vi "getWavelength_v80_AS1_actualTime.vi"() -> ()   [LabVIEW 2016]
uses:
  <vilib>/Analysis/baseanly.llb/Mean (DBL).vi
  <vilib>/Analysis/NI_AALBase.lvlib
  x32/CLDevIFace.dll
panel:
  out "Wavelength vs. time":dbl(graph)
  out "Wavelength":dbl format="%0.5f"
  out "0.75ppm in Wave (nm)":dbl format="%#_3g"
  out "0.75ppm in Freq (MHz)":dbl
  out "Freq (Hz)":dbl
  in  "Avg":i32=1
  out "Power (mW)":dbl format="%.9f"
  in  "Delay Time (s)":dbl=0.01
  out "error out":errorcluster
  out "output param":i32
  in  "stop":bool
  in  "OK Button":bool
  in  "CommPort":dbl=5.0 caption="Comm Port #"
  # "Pr = 605.977 nm"
  # "Super cavity FSR  6 GHz\nZerodure FSR  750 MHz"
  # "1 pm = 200 MHz @1212nm\n1 pm = 800 MHz @606 nm"
  # "Bristol 621B accuracy = 0.75 ppm\nuseful conversions:"
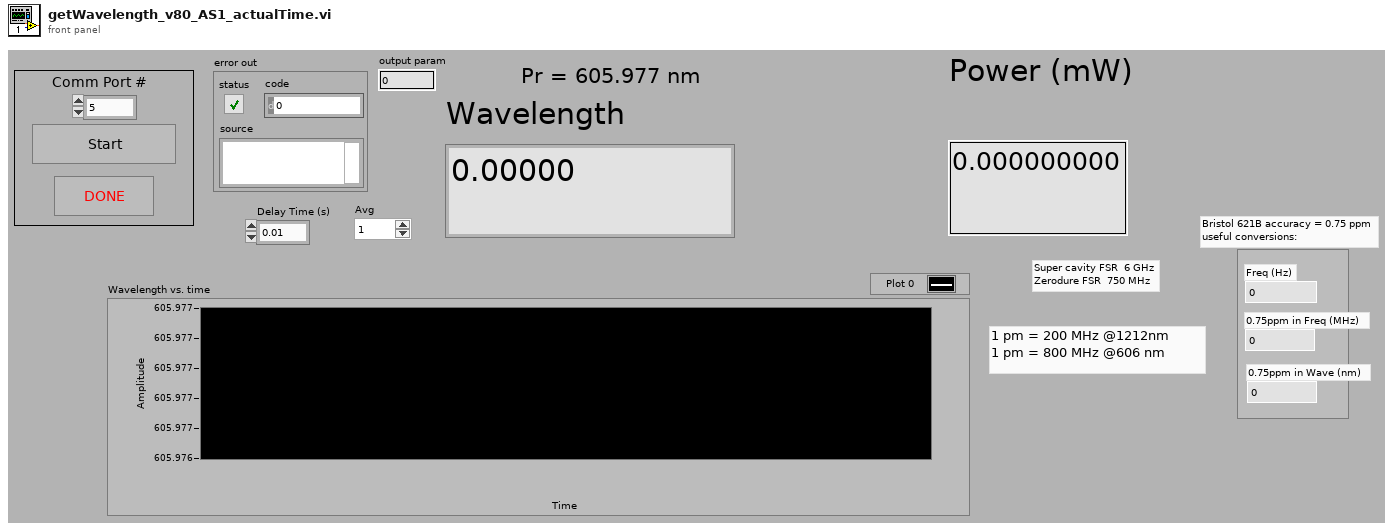
[diagram p1: front panel]
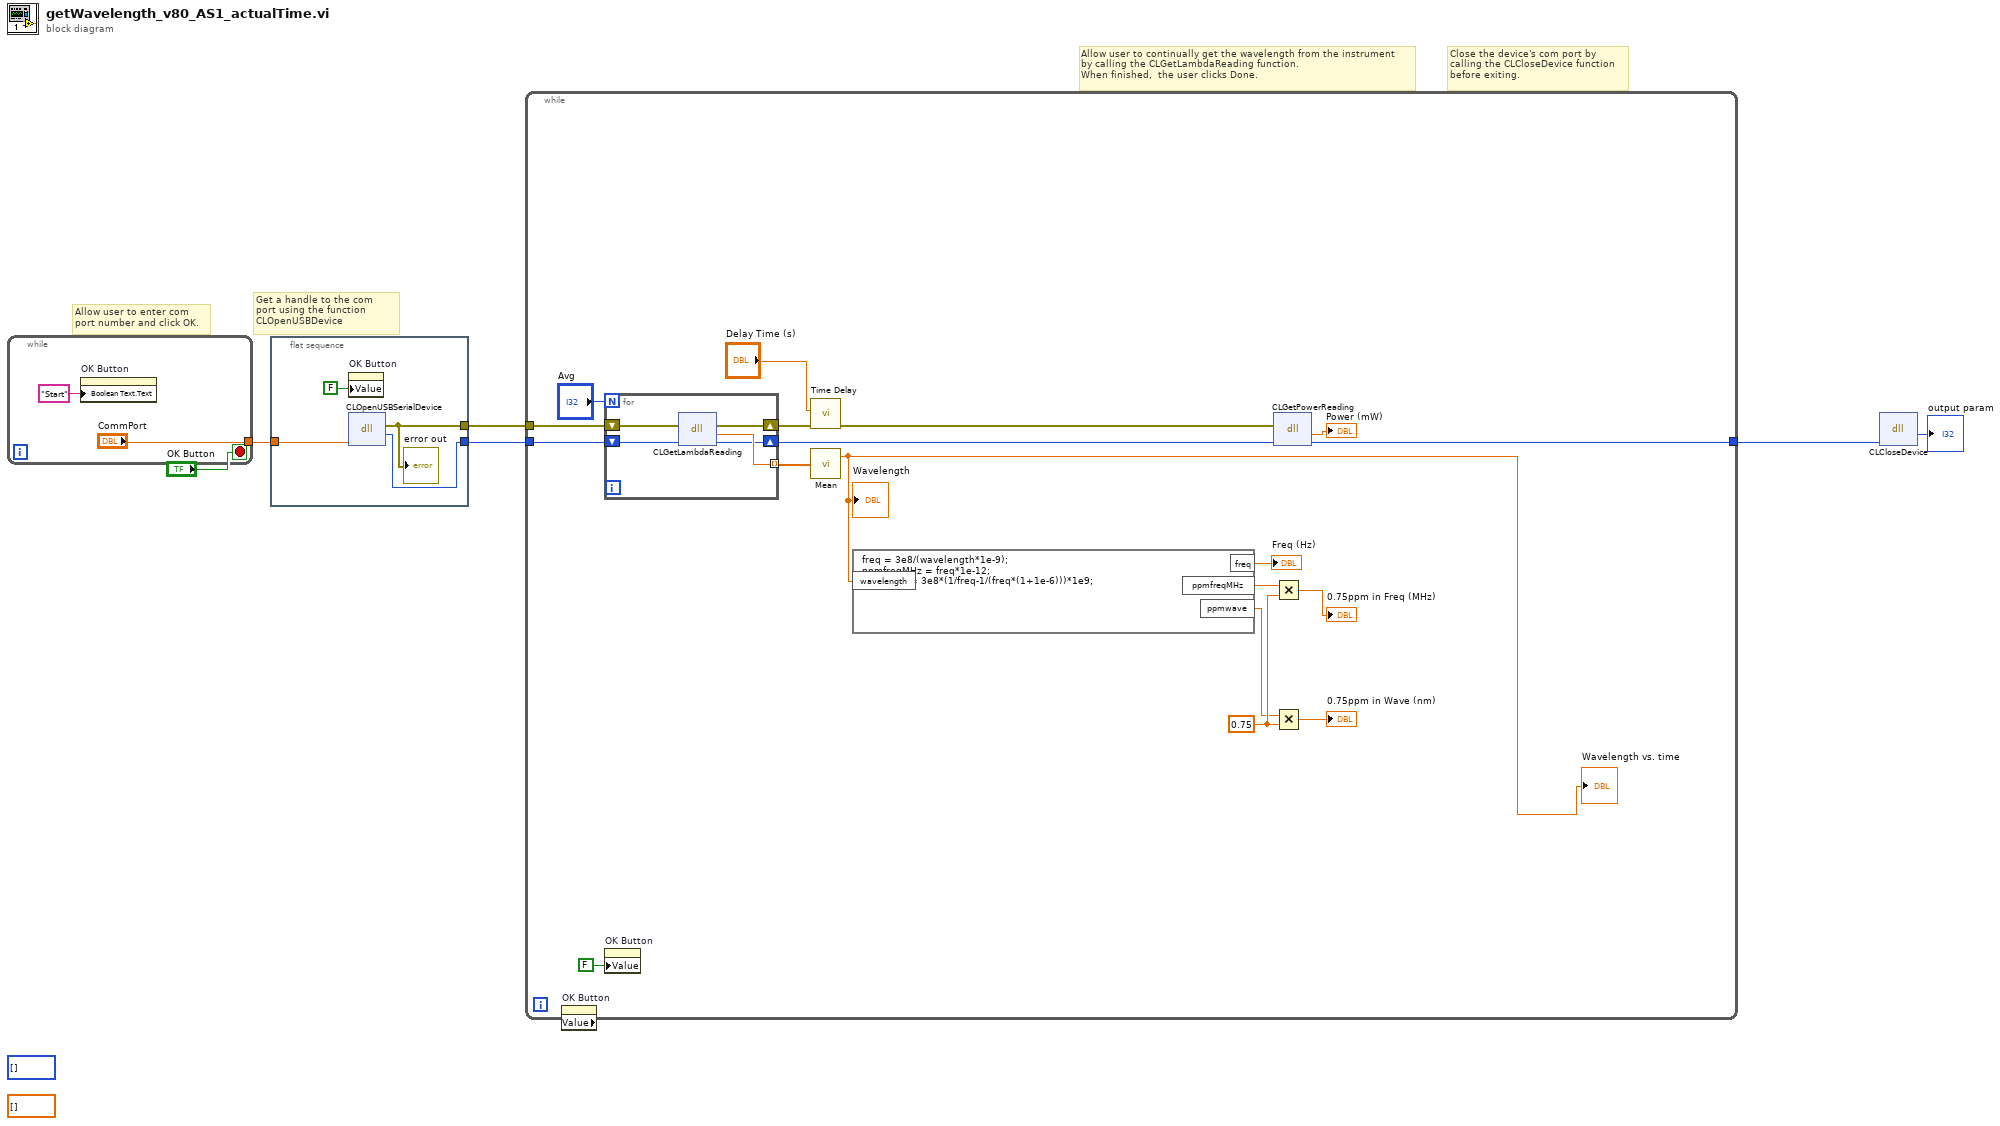
[diagram p0: block diagram]
diagram:
  (unwired) i32[] []
  (unwired) dbl[] []
  # "Close the device's com port by\ncalling the CLCloseDevice function\nbefore exiting."
  # "Allow user to continually get the wavelength from the instrument\nby calling the CLGetLambdaReading function.  \nWhen finished,  the user clicks Done."
  # "Get a handle to the com\nport using the function CLOpenUSBDevice"
  # "Allow user to enter com \nport number and click OK."
  n1 = while {
    tunnel: ["CommPort"] -> w5
    stop <- "OK Button" stop-if-true
    n2 = property on="OK Button" class="Bool (strict)"("Boolean Text.Text"="Start") -> ()  [unwired: 2 in, 2 out]
  }
  n3 = flat-sequence {
    tunnel: w5 -> [w12]
    tunnel: [w11] -> w4
    tunnel: [w9] -> w1
    frame #0 {
      n4 = property on="OK Button" class="Bool (strict)"("Value"=FALSE) -> ()  [unwired: 2 in, 2 out]
      n5 = dll-call lib="C:/Users/Lab/Desktop/Bristol wavemeter 621/00424-2-00 621 customer CD/Programming Interface/x32/CLDevIFace.dll" fn="CLOpenUSBSerialDevice"("commPort"=w12) -> (error out=w9:errorcluster, "return type"=w11:i32)  [unwired: 4 in, 1 out]
      "error out" <- w9
    }
  }
  n6 = while {
    tunnel: w4 -> [w31]
    tunnel: [w22] -> w3
    tunnel: w1 -> [w26]
    stop <- "stop" stop-if-true
    w16 = 0.75 ("y")
    n7 = property on="OK Button" class="Bool (strict)" props=["Value"]() -> ()  [unwired: 2 in, 3 out]
    n8 = for {
      N: "Avg" -> [_]
      tunnel: [w35] -> w20 mode=indexing
      shift-right: [w32] -> w23
      shift-left: w31 -> [w36]
      shift-right: [w34] -> w27
      shift-left: w26 -> [w33]
      n9 = dll-call lib="C:/Users/Lab/Desktop/Bristol wavemeter 621/00424-2-00 621 customer CD/Programming Interface/x32/CLDevIFace.dll" fn="CLGetLambdaReading"(error in=w33, "devHandle"=w36) -> (error out=w34:errorcluster, "return type"=w35:dbl, "devHandle"=w32:i32)  [unwired: 2 in, 1 out]
    }
    n10 = property on="OK Button" class="Bool (strict)"("Value"=FALSE) -> ()  [unwired: 2 in, 2 out]
    n11 = call "Time Delay"("error in (no error)"=w27, "Delay Time (s)"="Delay Time (s)") -> ("error out"=w25:errorcluster)  [unwired: 9 in]
    n12 = call-poly <vilib>:"Mean.vi"("X"=w20) -> ("mean"=w13:dbl)  [unwired: 1 out]
    "Wavelength" <- w13
    "Wavelength vs. time" <- w13
    n13 = formula code="freq = 3e8/(wavelength*1e-9);\nppmfreqMHz = freq*1e-12;\nppmwave = 3e8*(1/freq-1/(freq*(1+1e-6)))*1e9;"("wavelength"=w13) -> ("freq"=→"Freq (Hz)":dbl, "ppmfreqMHz"=w18:dbl, "ppmwave"=w15:dbl)
    n14 = dll-call lib="C:/Users/Lab/Desktop/Bristol wavemeter 621/00424-2-00 621 customer CD/Programming Interface/x32/CLDevIFace.dll" fn="CLGetPowerReading"(error in=w25, "devHandle"=w23) -> ("return type"=→"Power (mW)":dbl, "devHandle"=w22:i32)  [unwired: 2 in, 2 out]
    n15 = Multiply(x=w18, y=w16) -> (x*y=→"0.75ppm in Freq (MHz)":dbl)
    n16 = Multiply(x=w15, y=w16) -> (x*y=→"0.75ppm in Wave (nm)":dbl)
  }
  n17 = dll-call lib="C:/Users/Lab/Desktop/Bristol wavemeter 621/00424-2-00 621 customer CD/Programming Interface/x32/CLDevIFace.dll" fn="CLCloseDevice"("commPort"=w3) -> ("return type"=→"output param":i32)  [unwired: 4 in, 2 out]
